vi "Move Away from Framework and Back.vi"(8 "error in":errorcluster, 11 "Node Ptr in":T1 format="%.0x") -> (0 "error out":errorcluster)   [LabVIEW 2021, in "DSF System Explorer.lvlib"]
uses:
  DSF System Explorer.lvlib
  <vilib>/NI VeriStand/Custom Device API/Custom Device Item Ref.ctl
  <vilib>/NI VeriStand/Custom Device Tools/Custom Device Utility Library/Custom Device Utility Library.lvlib
  <vilib>/NI VeriStand/Custom Device Tools/Custom Device Utility Library/NI VeriStand - Search for Item by GUID.vi
  Shared/DSF Shared.lvlib
  <vilib>/NI VeriStand/Custom Device API/Custom Device API.lvlib
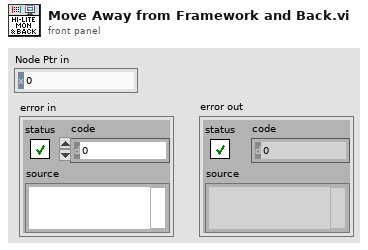
[diagram p1: front panel]
types:
  T1 = typedef "Custom Device API.lvlib/Custom Device Item Ref.ctl" = u64
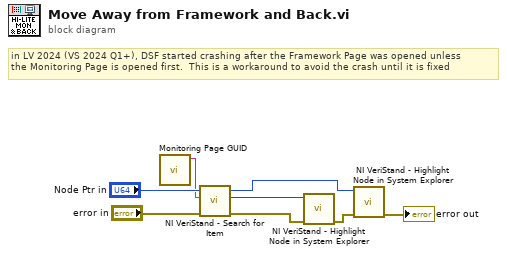
[diagram p0: block diagram]
diagram:
  # "in LV 2024 (VS 2024 Q1+), DSF started crashing after the Framework Page was opened unless \nthe Monitoring Page is opened first.  This is a workaround to avoid the crash until it is fixed"
  n1 = call "Monitoring Page GUID.vi"() -> ("Monitoring GUID"=w1:string)  [unwired: 11 in]
  n2 = call-poly <vilib>:"NI VeriStand - Search for Item.vi"("error in"="error in", "Item GUID"=w1, "Section Ref in"="Node Ptr in") -> ("error out"=w4:errorcluster, "Item Ref"=w5:T1, "Section Ref out"=w2:T1)  [unwired: 5 in, 1 out]
  n3 = call <vilib>:"NI VeriStand - Highlight Node in System Explorer.vi"("error in (no error)"=w4, "Item Ref in"=w5) -> ("error out"=w3:errorcluster)  [unwired: 8 in, 1 out]
  n4 = call <vilib>:"NI VeriStand - Highlight Node in System Explorer.vi"("error in (no error)"=w3, "Item Ref in"=w2) -> ("error out"=→"error out":errorcluster)  [unwired: 8 in, 1 out]
